vi "TimeKickForceIRL.vi"(8 "error in (no error)":errorcluster, 11 "Game in":refnum<class "Game.lvclass">) -> (0 "error out":errorcluster, 3 "Game out":refnum<class "Game.lvclass">)   [LabVIEW 2021, in "Game.lvclass"]
uses:
  Game.lvclass
panel:
  in  "RobotStopKick":bool
  out "Time":dbl
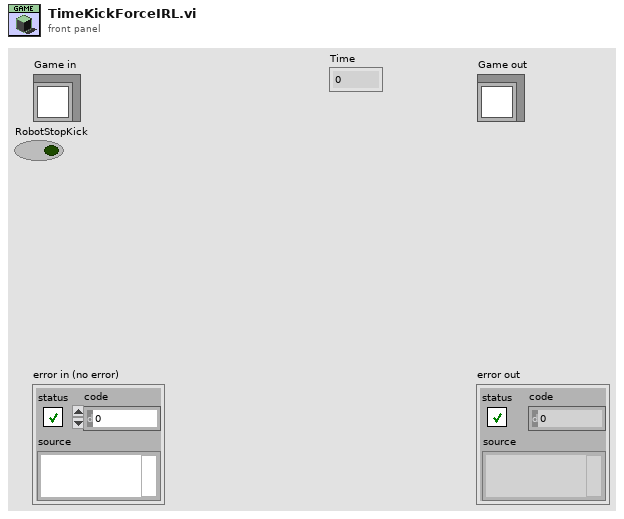
[diagram p1: front panel]
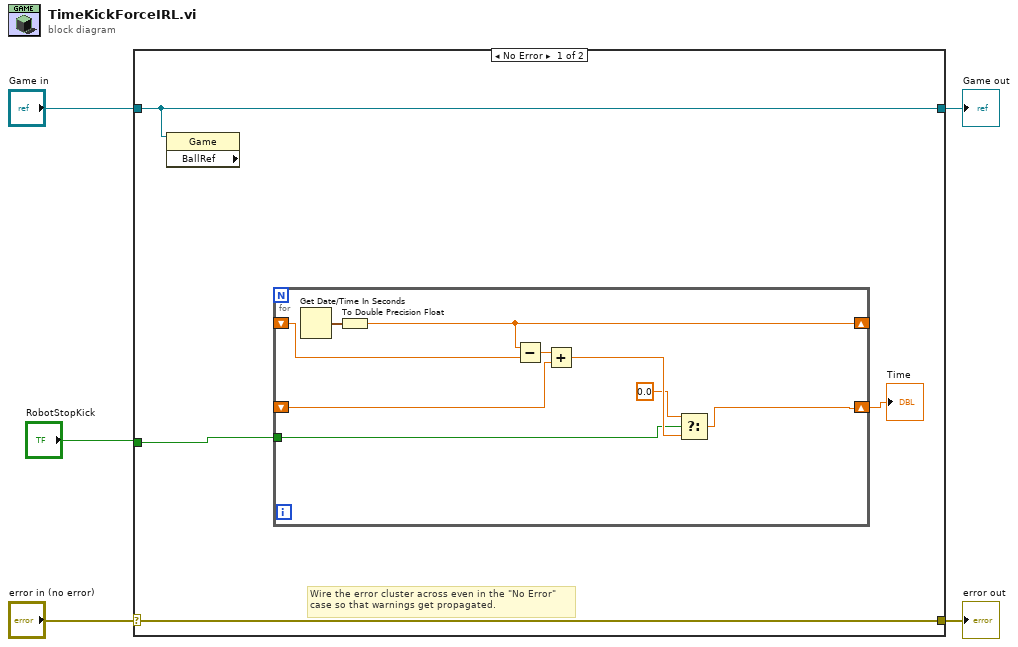
[diagram p0: block diagram]
diagram:
  n1 = case shown="No Error" "error in (no error)" {
    selector: "error in (no error)" -> [w9 w20]
    tunnel: [w9 w20] -> w4
    tunnel: [w8 w19] -> w2
    tunnel: "Game in" -> [w8 w19]
    tunnel: "RobotStopKick" -> [w6 _]
    frame No Error {
      # "Wire the error cluster across even in the \"No Error\"\ncase so that warnings get propagated."
      n2 = property class="Game" props=["BallRef"](reference=w8) -> ()  [unwired: 1 in, 3 out]
      n3 = for {
        shift-right: [w15] -> _
        shift-left: _ -> [w17]
        shift-right: [w12] -> w7
        shift-left: _ -> [w14]
        tunnel: w6 -> [w10]
        n4 = Get Date/Time In Seconds() -> (seconds since 1Jan1904=w18:timestamp)
        n5 = To Double Precision Float(number=w18) -> (double precision float=w15:dbl)
        n6 = Subtract(x=w15, y=w17) -> (x-y=w16:dbl)
        n7 = Add(x=w16, y=w14) -> (x+y=w13:dbl)
        n8 = Select(t=0.0, s=w10, f=w13) -> (s? t:f=w12:dbl)
      }
      "Time" <- w7
    }
    frame Error {
    }
  }
  "error out" <- w4
  "Game out" <- w2
